vi "Get all Object Item Offsets.vi"(8 "error in (no error)":errorcluster, 10 "Offset":i32, 11 "JSON":string) -> (0 "error out":errorcluster, 1 "Items":T1[](array[typedef]), 2 "Offset past Object":i32)   [LabVIEW 2017, in "JSONtext.lvlib"]
uses:
  JSONtext.lvlib
  Parsing/Found Items.ctl
  Parsing/Parsing State.ctl
  Parsing/Advance past Number.vi
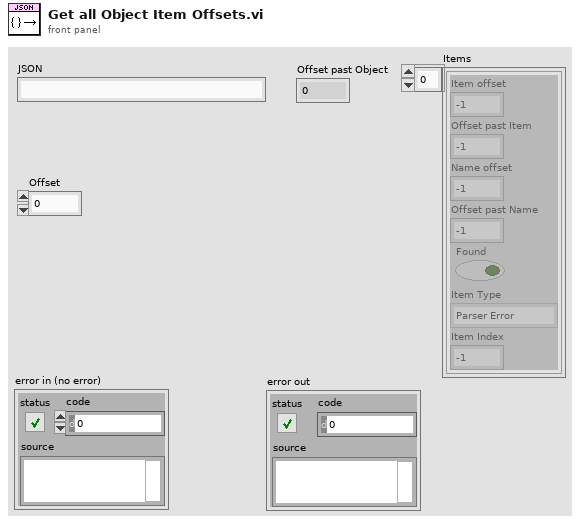
[diagram p1: front panel]
types:
  T1 = typedef "JSONtext.lvlib/Found Items.ctl" = cluster{"Item offset":i32, "Offset past Item":i32, "Name offset":i32, "Offset past Name":i32, "Found":bool, "Item Type":T2, "Item Index":i32}
  T2 = typedef "JSONtext.lvlib/Parsing State.ctl" = enum16{"Parser Error", "Object", "Array", "String", "Number/Other", "Leading Whitespace", "Object end", "Array end", "Value end"}
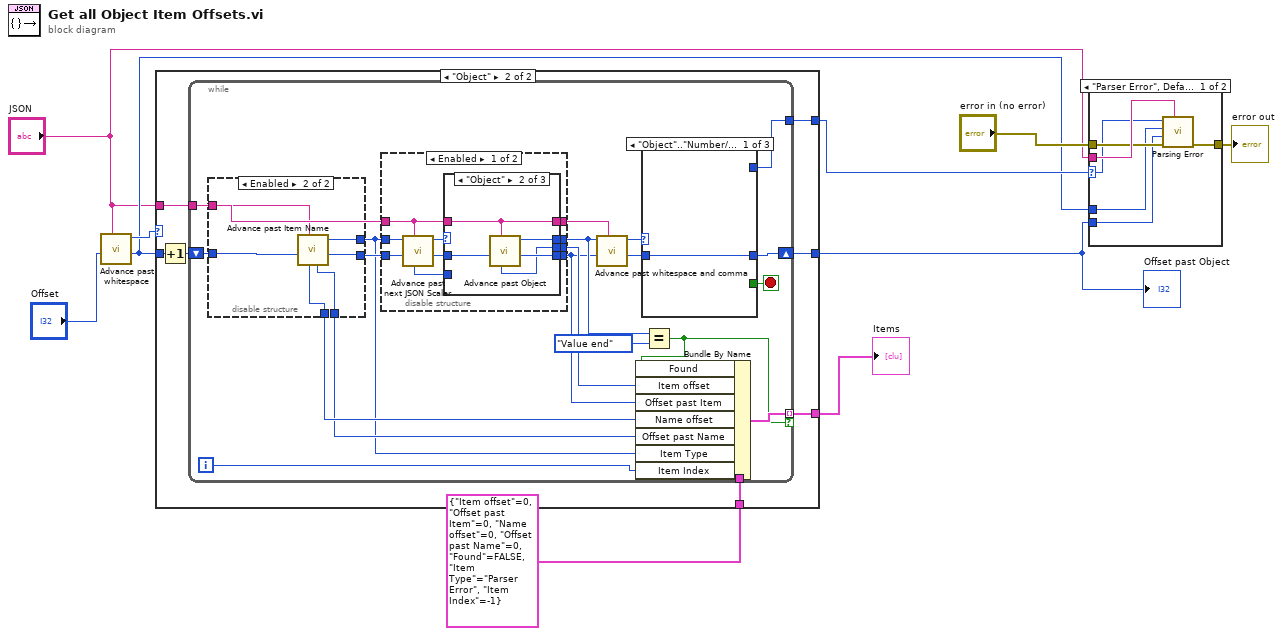
[diagram p0: block diagram]
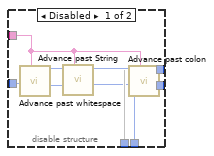
[diagram p4: hidden frame]
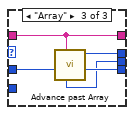
[diagram p6: hidden frame]
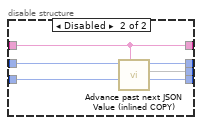
[diagram p7: hidden frame]
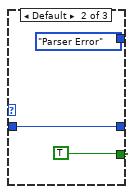
[diagram p8: hidden frame]
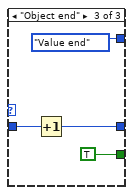
[diagram p9: hidden frame]
diagram:
  n1 = call "Advance past whitespace.vi"("JSON"="JSON", "Offset"="Offset") -> ("Offset of first non-whitespace"=w4:i32, "Parser State"=w9:T2)  [unwired: 8 in]
  n2 = case shown="\"Object\"" w9 {
    selector: w9 -> [w12 _]
    tunnel: [w12 w19] -> w5
    tunnel: w4 -> [w11 w17]
    tunnel: "JSON" -> [_ w16]
    tunnel: [w11 w15] -> w6
    tunnel: [_ w14] -> w2
    tunnel: T1 {"Item offset"=0, "Offset past Item"=0, "Name offset"=0, "Offset past Name"=0, "Found"=FALSE, "Item Type"=enum."Parser Error", "Item Index"=-1} -> [_ w13]
    frame "Parser Error", Default {
    }
    frame "Object" {
      n3 = Increment(x=w17) -> (x+1=w18:i32)
      n4 = while {
        shift-right: [w37] -> w15
        shift-left: w18 -> [w34]
        tunnel: w16 -> [w31]
        tunnel: [w35] -> w19
        tunnel: [w26] -> w14 mode=indexing if=w25
        tunnel: w13 -> [w22]
        i -> [w20]
        stop <- w36 stop-if-true
        n5 = disable-structure shown="Enabled" {
          disable-tunnel: w34 -> [w47 w52]
          disable-tunnel: [w44 w54] -> w21
          disable-tunnel: [w43 w53] -> w32
          disable-tunnel: w31 -> [w42 w51]
          disable-tunnel: [w41 w50] -> w24
          disable-tunnel: [w40 w49] -> w23
          frame Disabled {
            n6 = call "Advance past whitespace.vi"("JSON"=w42, "Offset"=w47) -> ("Offset of first non-whitespace"=w46:i32, "Parser State"=w45:T2)  [unwired: 8 in]
            n7 = call "Advance past String.vi"("JSON"=w42, "Offset"=w46, "State in"=w45) -> ("Offset past match"=w40:i32, 2:w41, "State"=w48:T2)  [unwired: 5 in, 1 out]
            n8 = call "Advance past colon.vi"("JSON"=w42, "Offset"=w40, "State"=w48) -> ("index"=w43:i32, "State"=w44:T2)  [unwired: 7 in]
          }
          frame Enabled {
            n9 = call "Advance past Item Name.vi"("JSON"=w51, "Offset"=w52) -> ("Offset past colon"=w53:i32, "State"=w54:T2, "Offset past Name"=w49:i32, "Name start out"=w50:i32)  [unwired: 6 in]
          }
        }
        n10 = disable-structure shown="Enabled" {
          disable-tunnel: [w64 w79] -> w33
          disable-tunnel: w21 -> [w62 w81]
          disable-tunnel: w32 -> [w61 w80]
          disable-tunnel: w31 -> [w59 w79]
          disable-tunnel: [w58 w82] -> w30
          disable-tunnel: [w57 w83] -> w28
          disable-tunnel: [w56 w84] -> w27
          frame Enabled {
            n11 = call "Advance past next JSON Scaler.vi"("JSON"=w59, "Offset"=w61, "Parser State in"=w62) -> ("index"=w60:i32, "Parser State"=w63:T2, "Value start"=w55:i32)  [unwired: 6 in]
            n12 = case shown="\"Object\"" w63 {
              selector: w63 -> [w67 _ _]
              tunnel: w60 -> [w66 w73 w78]
              tunnel: [w67 w72 w77] -> w58
              tunnel: [w66 w71 w76] -> w56
              tunnel: w59 -> [w68 w70 w75]
              tunnel: [w68 w70 w75] -> w64
              tunnel: [w65 w69 w74] -> w57
              tunnel: w55 -> [w65 _ _]
              frame Default {
              }
              frame "Object" {
                n13 = call "Advance past Object.vi"("JSON"=w70, "Offset"=w73) -> ("Offset past Object"=w71:i32, "State"=w72:T2, "Object Start"=w69:i32)  [unwired: 7 in]
              }
              frame "Array" {
                n14 = call "Advance past Array.vi"("JSON"=w75, "Offset"=w78) -> ("Offset past Array"=w76:i32, "State"=w77:T2, "Array Start"=w74:i32)  [unwired: 7 in]
              }
            }
          }
          frame Disabled {
            n15 = call "Advance past next JSON Value (inlined COPY).vi"("JSON"=w79, "Offset"=w80, "State"=w81) -> ("Offset"=w84:i32, 2:w83, "State"=w82:T2)  [unwired: 3 in, 3 out]
          }
        }
        n16 = call "Advance past whitespace and comma.vi"("JSON"=w33, "Offset"=w27, "State in"=w30) -> ("Offset past match"=w39:i32, "State"=w38:T2)  [unwired: 7 in]
        n17 = case shown="\"Object\"..\"Number/Other\"" w38 {
          tunnel: [_ TRUE TRUE] -> w36
          tunnel: [_ Parsing_State."Parser Error" Parsing_State."Value end"] -> w35
          tunnel: w39 -> [w85 w86 w90]
          tunnel: [w85 w86 w89] -> w37
          frame "Object".."Number/Other" {
          }
          frame Default {
          }
          frame "Object end" {
            n18 = Increment(x=w90) -> (x+1=w89:i32)
          }
        }
        n19 = Equal?(x=w30, y=Parsing_State."Value end") -> (x = y?=w25:bool)
        n20 = Bundle By Name(cluster=w22, "Found"=w25, "Item offset"=w28, "Offset past Item"=w27, "Name offset"=w24, "Offset past Name"=w23, "Item Type"=w21, "Item Index"=w20) -> (w26:T1)
      }
    }
  }
  "Offset past Object" <- w6
  "Items" <- w2
  n21 = case shown="\"Parser Error\", Default" w5 {
    selector: w5 -> [w93 _]
    tunnel: "JSON" -> [w98 _]
    tunnel: "error in (no error)" -> [w97 w99]
    tunnel: [w96 w99] -> w8
    tunnel: w4 -> [w95 _]
    tunnel: w6 -> [w94 _]
    frame "Parser Error", Default {
      n22 = call "Parsing Error.vi"("JSON"=w98, "error in (no error)"=w97, "Offset past match"=w94, "Value start"=w95, "State"=w93) -> ("error out"=w96:errorcluster)  [unwired: 6 in]
    }
    frame "Value end" {
    }
  }
  "error out" <- w8
